vi "Use case.vi"() -> ()   [LabVIEW 2024]
uses:
  SN Validator/SN Validator.lvlib
  <vilib>/TABOADA/Config File Management/Config Files Management/Config Files Management.lvlib
  SN Validator/SN_length.ctl
  SN Validator/SN_validation_mode.ctl
  SN Validator/SN_device_type.ctl
  SN Validator/SN_device_type_out.ctl
  SN Validator/SN Data.ctl
panel:
  out "SN Data":T1
  out "error out":errorcluster
  in  "Device Type":T3
  in  "Parse mode":T4
  in  "Length range":T5
  in  "Serial Number in":string
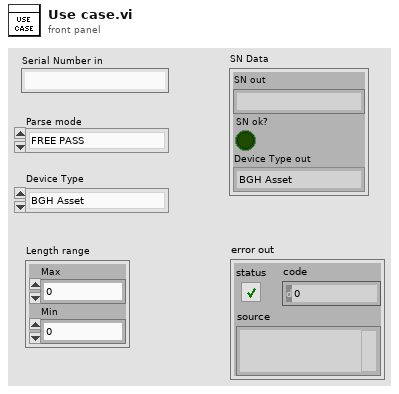
[diagram p1: front panel]
types:
  T1 = typedef "SN Validator.lvlib/SN Data.ctl" = cluster{"SN out":string, "SN ok?":bool, "Device Type out":T2}
  T2 = typedef "SN Validator.lvlib/SN_device_type_out.ctl" = enum16{"BGH Asset", "BGH Product", "SAMSUNG Product", "GENERIC Product", "No Product", ""}
  T3 = typedef "SN Validator.lvlib/SN_device_type.ctl" = enum16{"BGH Asset", "BGH Product", "SAMSUNG Product"}
  T4 = typedef "SN Validator.lvlib/SN_validation_mode.ctl" = enum16{"FREE PASS", "LENGTH BASED", "REGEX BASED", "AUTO"}
  T5 = typedef "SN Validator.lvlib/SN_length.ctl" = cluster{"Max":i32, "Min":i32}
  T6 = typedef "NI_LVConfig.lvlib/Config Data RefNum.ctl" = refnum<k1>
  T7 = typedef "Config Files Management.lvlib/config data--cluster.ctl" = cluster{"sections":string[][], "key names":string[], "values":string[]}
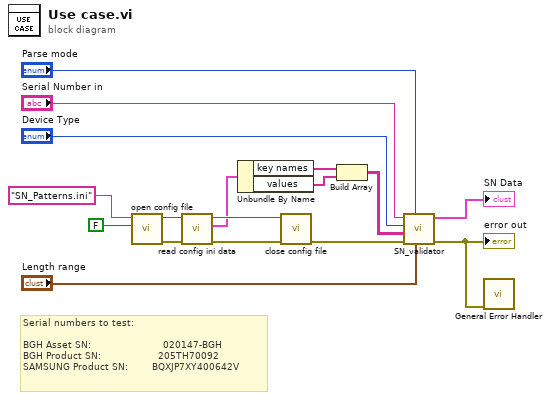
[diagram p0: block diagram]
diagram:
  # "Serial numbers to test: \n\nBGH Asset SN:                        020147-BGH\nBGH Product SN:                   205TH70092\nSAMSUNG Product SN:        BQXJP7XY400642V"
  n1 = call <vilib>:"open config file.vi"("create file if necessary (T)"=FALSE, "file name"="SN_Patterns.ini") -> ("error out"=w8:errorcluster, "Refnum out"=w7:T6)  [unwired: 7 in, 1 out]
  n2 = call <vilib>:"read config ini data.vi"("error in (no error)"=w8, "Refnum in"=w7) -> ("error out"=w6:errorcluster, "data out"=w3:T7, "Refnum out"=w4:T6)  [unwired: 7 in]
  n3 = Unbundle By Name(w3) -> ("key names"=w17:string[], "values"=w16:string[])
  n4 = call <vilib>:"close config file.vi"("error in (no error)"=w6, "Refnum in"=w4) -> ("error out"=w5:errorcluster)  [unwired: 9 in]
  n5 = Build Array(w17, w16) -> (w15:string[][])
  n6 = call "SN_validator.vi"("Length range"="Length range", "Validaton mode"="Parse mode", "error in (no error)"=w5, "SN Regex"=w15, "Device Type"="Device Type", "SN in"="Serial Number in") -> ("error out"=w9:errorcluster, "SN Data"=→"SN Data":T1)  [unwired: 4 in]
  "error out" <- w9
  n7 = call <vilib>:"General Error Handler.vi"("error in (no error)"=w9) -> ()  [unwired: 10 in, 5 out]
